vi "Write Path.vi"(8 "error in (no error)":errorcluster, 10 "Path":path=path "C:/Users/public/Documents/Development/Application", 11 "Launcher in":refnum<class "Launcher.lvclass">) -> (0 "error out":errorcluster, 3 "Launcher out":refnum<class "Launcher.lvclass">)   [LabVIEW 2019, in "Launcher.lvlib" / "Launcher.lvclass"]
uses:
  Library/Launcher.lvclass
  Library/Launcher.lvclass/Launcher.ctl
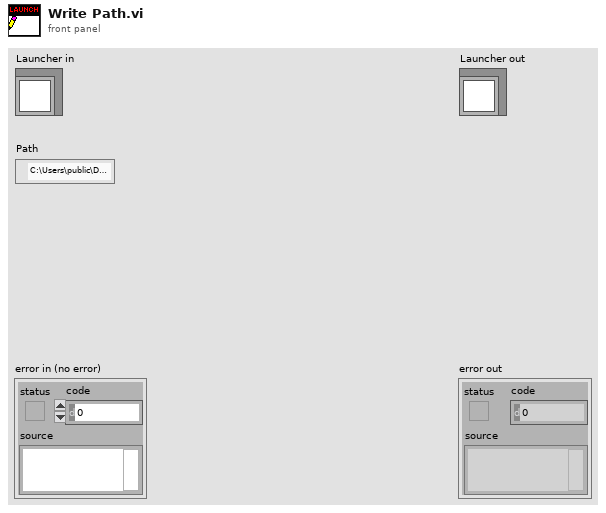
[diagram p1: front panel]
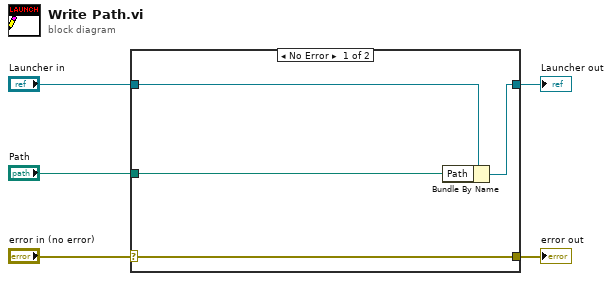
[diagram p0: block diagram]
diagram:
  n1 = case shown="No Error" "error in (no error)" {
    selector: "error in (no error)" -> [w9 w10]
    tunnel: [w9 w10] -> w4
    tunnel: [w7 w11] -> w2
    tunnel: "Launcher in" -> [w8 w11]
    tunnel: "Path" -> [w6 _]
    frame No Error {
      n2 = Bundle By Name(cluster=w8, "Path"=w6) -> (w7:refnum<class "Launcher.lvclass">)
    }
    frame Error {
    }
  }
  "error out" <- w4
  "Launcher out" <- w2
